vi "UpdateFlagState.vi"(8 "error in (no error)":errorcluster, 10 "FlagState":bool[](array[boolean])=[FALSE, FALSE, FALSE, FALSE], 11 "Room Number":i32) -> (0 "error out":errorcluster, 2 "Response":string)   [LabVIEW 2015, in "RoomRestApi.lvlib"]
uses:
  RoomRestApi.lvlib
  TypeDef/PostRoomCommands.ctl
panel:
  out "JSON string":string
  # "{\"FlagsState\":\"{\\\"State\\\":[false,false,false,false],\\\"Color\\\":[0,1,2,3]}\"}"
  # "http://127.0.0.1:8001/WebService1/UpdateFlagState?Room={value}&FlagState={value}"
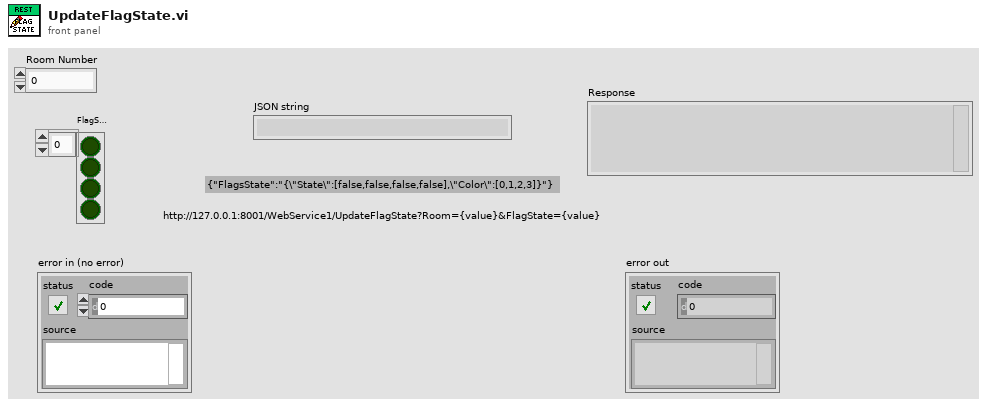
[diagram p1: front panel]
types:
  T1 = typedef "RoomRestApi.lvlib/PostRoomCommands.ctl" = enum16{"WriteFlagState", "WriteFlagColor", "WriteBedVacant", "AddPersonnel", "RemovePersonnel", "AddRequest", "RemoveRequest", "WriteBeaconID", "WriteBedURL", "WriteFlag"}
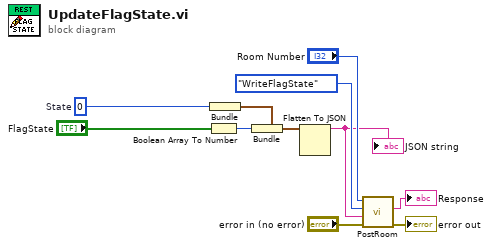
[diagram p0: block diagram]
diagram:
  w6 = u32 0  # State
  n1 = Boolean Array To Number(Boolean array="FlagState") -> (number=w5:u32)
  n2 = Bundle("State"=w6) -> (w4:cluster{"State":u32})  [unwired: 1 in]
  n3 = Bundle(cluster=w4, "State"=w5) -> (w3:cluster{"State":u32})
  n4 = Flatten To JSON(anything=w3) -> (JSON string=w2:string)  [unwired: 2 in, 1 out]
  "JSON string" <- w2
  n5 = call "PostRoom.vi"("error in (no error)"="error in (no error)", "Data"=w2, "Enum"=PostRoomCommands."WriteFlagState", "Room Number"="Room Number") -> ("error out"=→"error out":errorcluster, "body"=→"Response":string)  [unwired: 6 in]
